vi "torque_decluster_by_time.vi"(9 "t_final":dbl format="%_19f", 10 "t_init":dbl format="%_19f", 11 "torque array cluster":T1) -> (2 "Dados":dbl[][](array[numeric]), 3 "Tempo":dbl[](array[numeric]))   [LabVIEW 2019]
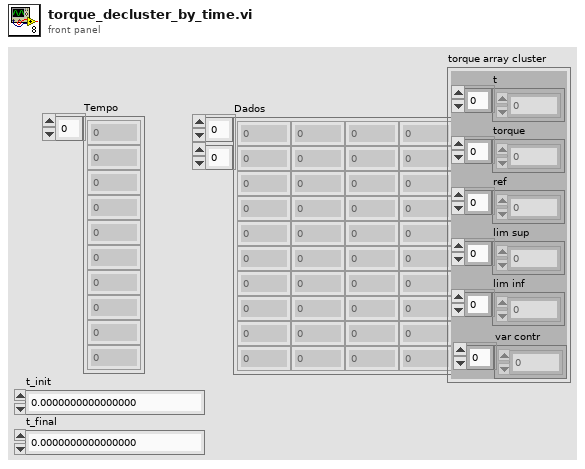
[diagram p1: front panel]
types:
  T1 = cluster{"t":dbl[], "torque":dbl[], "ref":dbl[], "lim sup":dbl[], "lim inf":dbl[], "var contr":dbl[]}
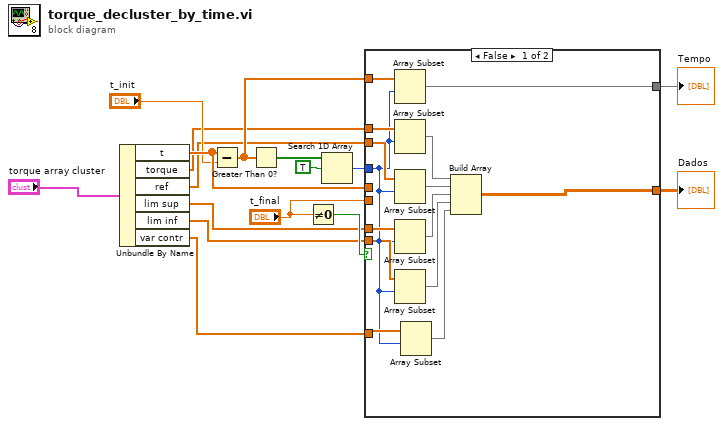
[diagram p0: block diagram]
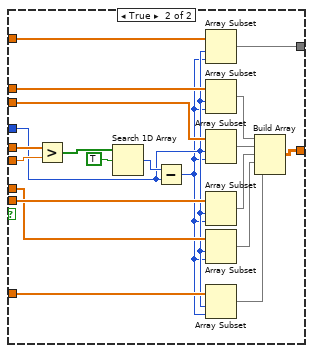
[diagram p2: hidden frame]
diagram:
  n1 = Unbundle By Name("torque array cluster") -> ("t"=w10:dbl[], "torque"=w4:dbl[], "ref"=w5:dbl[], "lim sup"=w7:dbl[], "lim inf"=w6:dbl[], "var contr"=w1:dbl[])
  n2 = Subtract(x=w10, y="t_init") -> (x-y=w13:dbl[])
  n3 = Greater Than 0?(x=w13) -> (x > 0?=w15:bool[])
  n4 = Not Equal To 0?(x="t_final") -> (x != 0?=w14:bool)
  n5 = Search 1D Array(1D array=w15, element=TRUE) -> (index of element=w12:i32)  [unwired: 1 in]
  n6 = case shown="False" w14 {
    tunnel: w13 -> [w30 w50]
    tunnel: w12 -> [w18 w32]
    tunnel: [w29 w49] -> w11
    tunnel: "t_final" -> [_ w45]
    tunnel: w10 -> [_ w44]
    tunnel: w7 -> [w24 w36]
    tunnel: w6 -> [w23 w37]
    tunnel: w5 -> [w22 w38]
    tunnel: w4 -> [w21 w39]
    tunnel: [w20 w35] -> w3
    tunnel: w1 -> [w19 w33]
    frame False {
      n7 = Array Subset(array=w30, index=w18) -> (w29:dbl[])  [unwired: 1 in]
      n8 = Array Subset(array=w21, index=w18) -> (w25:dbl[])  [unwired: 1 in]
      n9 = Array Subset(array=w22, index=w18) -> (w26:dbl[])  [unwired: 1 in]
      n10 = Array Subset(array=w24, index=w18) -> (w27:dbl[])  [unwired: 1 in]
      n11 = Array Subset(array=w23, index=w18) -> (w28:dbl[])  [unwired: 1 in]
      n12 = Array Subset(array=w19, index=w18) -> (w17:dbl[])  [unwired: 1 in]
      n13 = Build Array(w25, w26, w27, w28, w17) -> (w20:dbl[][])
    }
    frame True {
      n14 = Greater?(x=w44, y=w45) -> (0:w47:bool[])
      n15 = Search 1D Array(1D array=w47, element=TRUE) -> (index of element=w48:i32)  [unwired: 1 in]
      n16 = Subtract(x=w48, y=w32) -> (x-y=w31:i32)
      n17 = Array Subset(array=w50, index=w32, length=w31) -> (w49:dbl[])
      n18 = Array Subset(array=w39, index=w32, length=w31) -> (w40:dbl[])
      n19 = Array Subset(array=w38, index=w32, length=w31) -> (w41:dbl[])
      n20 = Array Subset(array=w37, index=w32, length=w31) -> (w42:dbl[])
      n21 = Array Subset(array=w36, index=w32, length=w31) -> (w43:dbl[])
      n22 = Array Subset(array=w33, index=w32, length=w31) -> (w34:dbl[])
      n23 = Build Array(w40, w41, w42, w43, w34) -> (w35:dbl[][])
    }
  }
  "Tempo" <- w11
  "Dados" <- w3
